vi "Device.Uninit.vi"(8 "error in (no error)":errorcluster, 11 "OPA.OrpheusHP in":refnum<class "OPA.OrpheusHP.lvclass">) -> (0 "error out":errorcluster, 3 "OPA.OrpheusHP out":refnum<class "OPA.OrpheusHP.lvclass">)   [LabVIEW 2017, in "OPA.OrpheusHP.lvclass"]
uses:
  OPA.OrpheusHP.lvclass
  OPA/OPA.lvclass
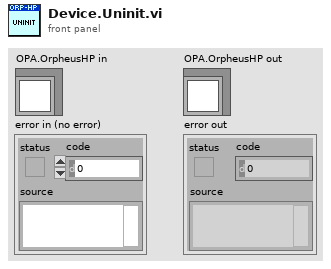
[diagram p1: front panel]
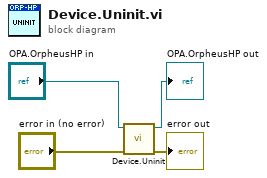
[diagram p0: block diagram]
diagram:
  n1 = call-parent "Device.Uninit.vi"("error in (no error)"="error in (no error)", "Device in"="OPA.OrpheusHP in") -> ("error out"=→"error out":errorcluster, "Device out"=→"OPA.OrpheusHP out":refnum<class "OPA.OrpheusHP.lvclass">)  [unwired: 8 in]
